vi "projetoIM_labview2021.vi"() -> ()   [LabVIEW 2020]
uses:
  <vilib>/express/express shared/transition.llb/Dynamic To Waveform Array.vi
  <vilib>/express/express arith-compare/Formula/Block/exnFormulaBlock how many pts in the wave.vi
  <vilib>/express/express shared/ex_Modify Signal Name.vi
  <vilib>/express/express shared/transition.llb/Waveform Array To Dynamic.vi
  <vilib>/express/express arith-compare/Formula/XNode/ExpressFormulaBlockNode.xnode
panel:
  in  "Interface":enum16{"R5.00", "R6.25"}(ring)
  in  "Rg":enum16{"3k3", "1k5"}(ring)
  out "Força":dbl(knob) scale=0.0..350.0
  out "R_fsr":dbl
  out "Força":dbl
  out "Vout":dbl
  in  "stop":bool
  out "data":dynamicdata(graph) caption="Vout"
  # "mm"
  # "ohm"
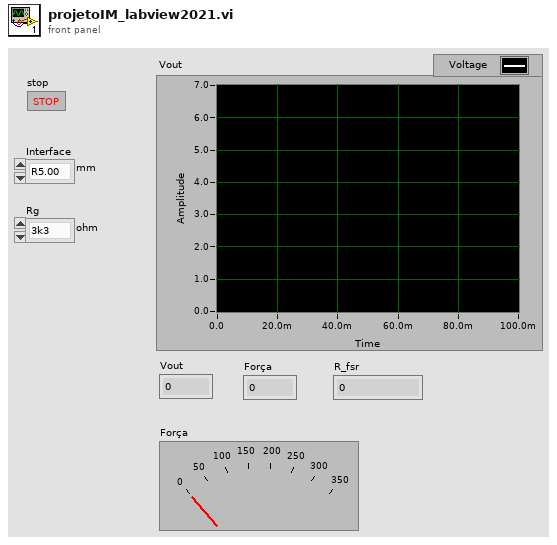
[diagram p1: front panel]
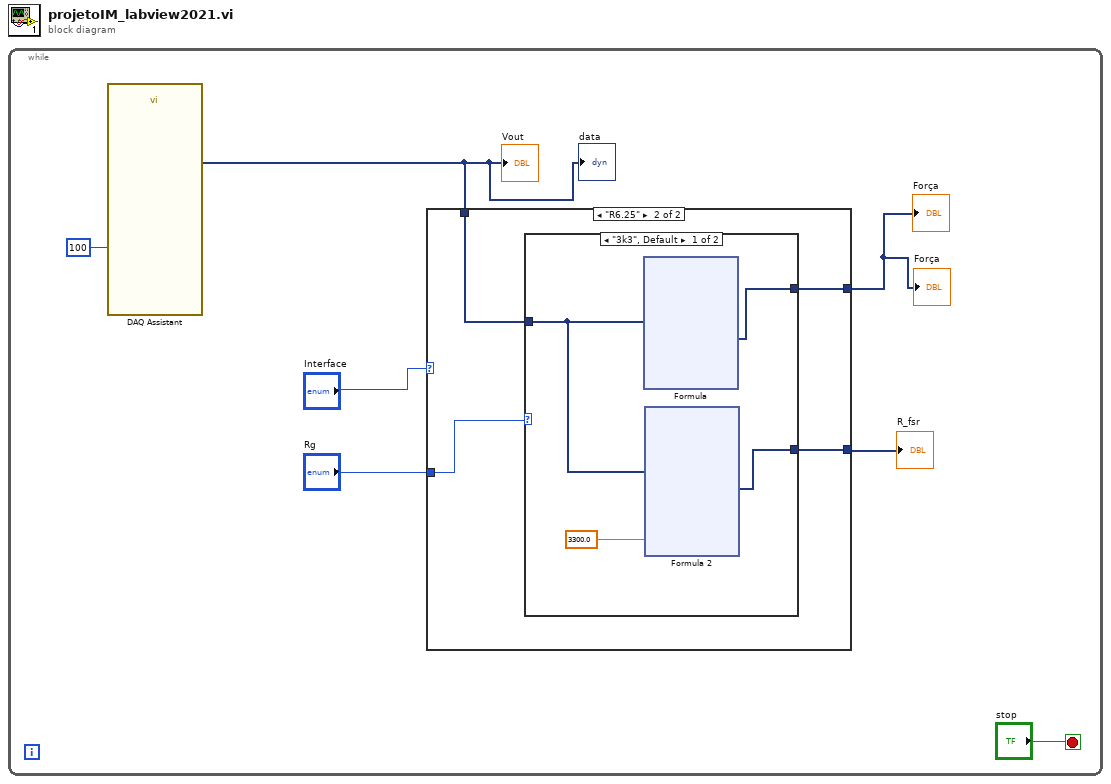
[diagram p0: block diagram]
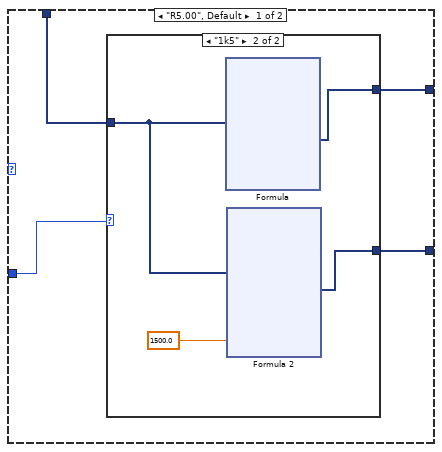
[diagram p2: hidden frame]
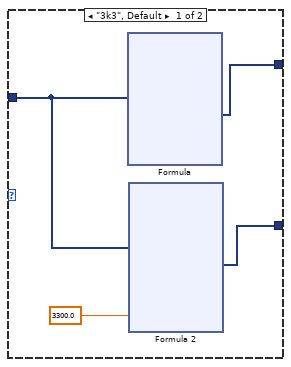
[diagram p3: hidden frame]
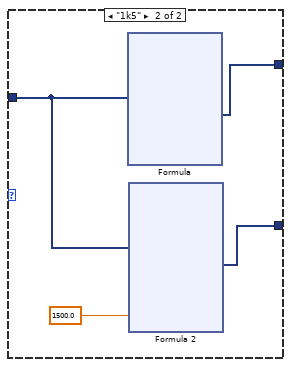
[diagram p4: hidden frame]
diagram:
  n1 = while {
    stop <- "stop" stop-if-true
    n2 = call "DAQ Assistant"("number of samples"=100) -> ("data"=w1:dynamicdata)  [unwired: 16 in, 2 out]
    "data" <- w1
    "Vout" <- w1
    n3 = case shown="\"R6.25\"" "Interface" {
      tunnel: w1 -> [w11 w579]
      tunnel: [w10 w578] -> w4
      tunnel: [w9 w577] -> w5
      tunnel: "Rg" -> [w8 w576]
      frame "R5.00", Default {
        n4 = case shown="\"1k5\"" w8 {
          tunnel: w11 -> [w15 w297]
          tunnel: [w14 w296] -> w10
          tunnel: [w13 w295] -> w9
          frame "3k3", Default {
            n5 = xnode "Formula"("X1"=w15) -> ("Result"=w14:dynamicdata)  [unwired: 1 in, 1 out]
            n6 = xnode "Formula 2"("X1"=w15, "X2"=3300.0) -> ("Result"=w13:dynamicdata)  [unwired: 1 in, 1 out]
          }
          frame "1k5" {
            n7 = xnode "Formula"("X1"=w297) -> ("Result"=w296:dynamicdata)  [unwired: 1 in, 1 out]
            n8 = xnode "Formula 2"("X1"=w297, "X2"=1500.0) -> ("Result"=w295:dynamicdata)  [unwired: 1 in, 1 out]
          }
        }
      }
      frame "R6.25" {
        n9 = case shown="\"3k3\", Default" w576 {
          tunnel: w579 -> [w583 w865]
          tunnel: [w582 w864] -> w578
          tunnel: [w581 w863] -> w577
          frame "3k3", Default {
            n10 = xnode "Formula"("X1"=w583) -> ("Result"=w582:dynamicdata)  [unwired: 1 in, 1 out]
            n11 = xnode "Formula 2"("X1"=w583, "X2"=3300.0) -> ("Result"=w581:dynamicdata)  [unwired: 1 in, 1 out]
          }
          frame "1k5" {
            n12 = xnode "Formula"("X1"=w865) -> ("Result"=w864:dynamicdata)  [unwired: 1 in, 1 out]
            n13 = xnode "Formula 2"("X1"=w865, "X2"=1500.0) -> ("Result"=w863:dynamicdata)  [unwired: 1 in, 1 out]
          }
        }
      }
    }
    "Força" <- w4
    "R_fsr" <- w5
    "Força" <- w4
  }
